vi "Elapsed Time.vi"(1 "Start Timing(ms)":u32) -> (0 "Elapsed Time(s)":dbl)   [LabVIEW 2024]
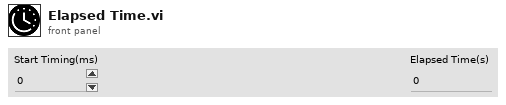
[diagram p1: front panel]
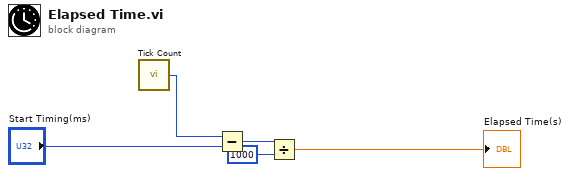
[diagram p0: block diagram]
diagram:
  n1 = call "Tick Count"() -> ("Tick Count(mSec)"=w5:u32)
  n2 = Subtract(x=w5, y="Start Timing(ms)") -> (x-y=w3:u32)
  n3 = Divide(x=w3, y=u32 1000) -> (x/y=→"Elapsed Time(s)":dbl)
